vi "OuputMixer5782_1Ghz_interpolated_single_cycle.vi"(6 "Standard interp":bool=TRUE, 7 "reset":bool, 8 "input valid":bool=TRUE, 9 "Sine in":fxp<+/-,16,0>[](array[numeric])=[0.0, 0.0, 0.0, 0.0], 10 "Cosine in":fxp<+/-,16,0>[](array[numeric])=[0.0, 0.0, 0.0, 0.0], 11 "Data":fxp<+/-,16,14>[](array[numeric])=[0.0, 0.0]) -> (3 "test":i16[](array[numeric]))   [LabVIEW 2018]
doc: "Outputs input from channel 0 as I*cos(t)-Q*sin(t) on analog output 0"
uses:
  <vilib>/rvi/eio/common/nirviEmuTemplateMethod_errors.vi
  <vilib>/eio/EIONode/EIONode.xnode
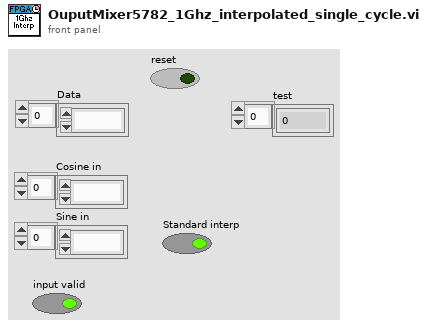
[diagram p1: front panel]
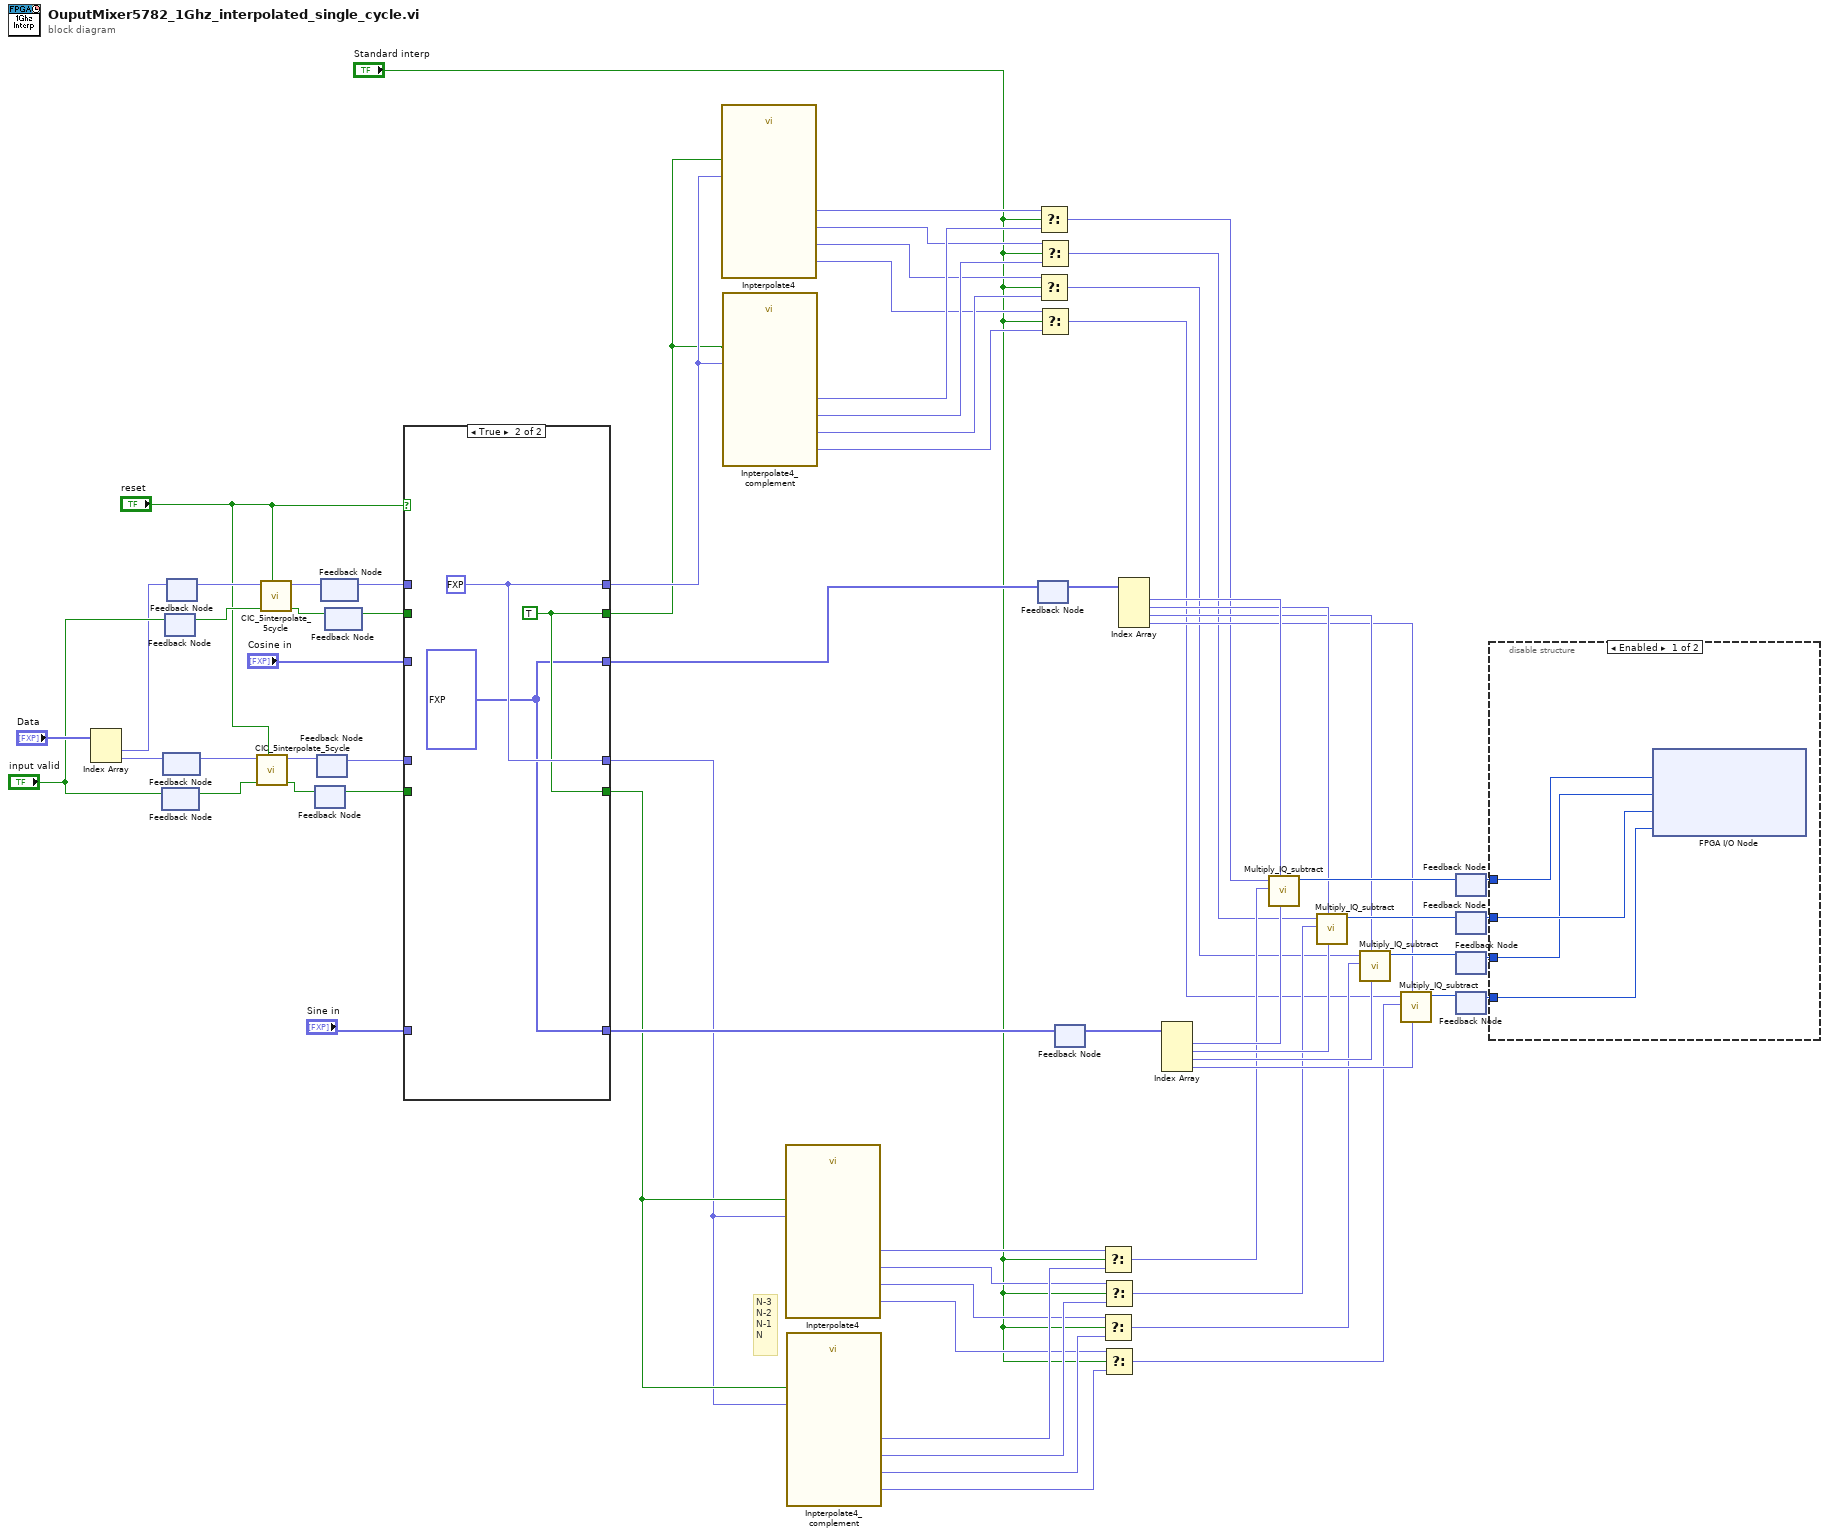
[diagram p0: block diagram]
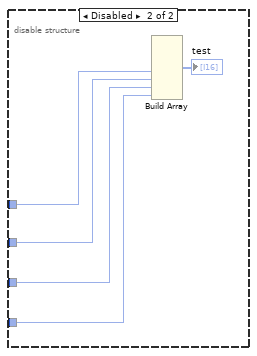
[diagram p3: hidden frame]
diagram:
  # "N-3\nN-2\nN-1\nN"
  n1 = Index Array(array="Data") -> (element #1=w46:fxp<+/-,16,14>, element #2=w47:fxp<+/-,16,14>)  [unwired: 2 in]
  n2 = feedback #1() -> (w54:bool)  [unwired: 1 in]
  n3 = feedback-in #1("input valid") -> ()
  n4 = feedback #2() -> (w56:fxp<+/-,16,14>)  [unwired: 1 in]
  n5 = feedback-in #2(w47) -> ()
  n6 = feedback #3() -> (w55:bool)  [unwired: 1 in]
  n7 = feedback-in #3("input valid") -> ()
  n8 = feedback #4() -> (w57:fxp<+/-,16,14>)  [unwired: 1 in]
  n9 = feedback-in #4(w46) -> ()
  n10 = call "CIC_5interpolate_5cycle.vi"("reset"="reset", "valid in"=w54, "Data in"=w56) -> ("valid out"=w48:bool, "Data out"=w53:fxp<+/-,16,14>)  [unwired: 7 in]
  n11 = call "CIC_5interpolate_5cycle.vi"("reset"="reset", "valid in"=w55, "Data in"=w57) -> ("valid out"=w49:bool, "Data out"=w52:fxp<+/-,16,14>)  [unwired: 7 in]
  n12 = feedback #5() -> (w35:bool)  [unwired: 1 in]
  n13 = feedback-in #5(w48) -> ()
  n14 = feedback #6() -> (w36:fxp<+/-,16,14>)  [unwired: 1 in]
  n15 = feedback-in #6(w53) -> ()
  n16 = feedback #7() -> (w32:fxp<+/-,16,14>)  [unwired: 1 in]
  n17 = feedback-in #7(w52) -> ()
  n18 = feedback #8() -> (w31:bool)  [unwired: 1 in]
  n19 = feedback-in #8(w49) -> ()
  n20 = case shown="True" "reset" {
    tunnel: [w71 w75] -> w66
    tunnel: w32 -> [w70 _]
    tunnel: "Cosine in" -> [w71 _]
    tunnel: w36 -> [w74 _]
    tunnel: [w74 w77] -> w28
    tunnel: w35 -> [w73 _]
    tunnel: [w73 w76] -> w29
    tunnel: "Sine in" -> [w72 _]
    tunnel: [w72 w75] -> w33
    tunnel: [w70 w77] -> w7
    tunnel: w31 -> [w69 _]
    tunnel: [w69 w76] -> w6
    frame False {
    }
    frame True {
      w75 = fxp<+/-,16,0>[] [0.0, 0.0, 0.0, 0.0] ("Cosine in")
      w76 = TRUE ("valid out")
      w77 = fxp<+/-,16,14> 0.0 ("Data out")
    }
  }
  n21 = call "Inpterpolate4.vi"("X"=w7, "input valid"=w6) -> ("X(t)"=w8:fxp<+/-,16,14>, "X(t -1)"=w9:fxp<+/-,16,14>, "X(t -2)"=w10:fxp<+/-,16,14>, "X(t -3)"=w11:fxp<+/-,16,14>)  [unwired: 9 in, 1 out]
  n22 = call "Inpterpolate4_complement.vi"("X"=w7, "input valid"=w6) -> ("X(t)"=w15:fxp<+/-,16,14>, "X(t -1)"=w13:fxp<+/-,16,14>, "X(t -2)"=w12:fxp<+/-,16,14>, "X(t -3)"=w14:fxp<+/-,16,14>)  [unwired: 9 in, 1 out]
  n23 = call "Inpterpolate4.vi"("X"=w28, "input valid"=w29) -> ("X(t)"=w16:fxp<+/-,16,14>, "X(t -1)"=w17:fxp<+/-,16,14>, "X(t -2)"=w18:fxp<+/-,16,14>, "X(t -3)"=w19:fxp<+/-,16,14>)  [unwired: 9 in, 1 out]
  n24 = call "Inpterpolate4_complement.vi"("X"=w28, "input valid"=w29) -> ("X(t)"=w27:fxp<+/-,16,14>, "X(t -1)"=w23:fxp<+/-,16,14>, "X(t -2)"=w22:fxp<+/-,16,14>, "X(t -3)"=w24:fxp<+/-,16,14>)  [unwired: 9 in, 1 out]
  n25 = feedback #9() -> (w67:fxp<+/-,16,0>[])  [unwired: 1 in]
  n26 = feedback-in #9(w66) -> ()
  n27 = Select(t=w11, s="Standard interp", f=w14) -> (s? t:f=w5:fxp<+/-,16,14>)
  n28 = Select(t=w9, s="Standard interp", f=w13) -> (s? t:f=w3:fxp<+/-,16,14>)
  n29 = Select(t=w10, s="Standard interp", f=w12) -> (s? t:f=w4:fxp<+/-,16,14>)
  n30 = Select(t=w8, s="Standard interp", f=w15) -> (s? t:f=w2:fxp<+/-,16,14>)
  n31 = feedback #10() -> (w68:fxp<+/-,16,0>[])  [unwired: 1 in]
  n32 = feedback-in #10(w33) -> ()
  n33 = Select(t=w19, s="Standard interp", f=w24) -> (s? t:f=w20:fxp<+/-,16,14>)
  n34 = Select(t=w17, s="Standard interp", f=w23) -> (s? t:f=w25:fxp<+/-,16,14>)
  n35 = Select(t=w18, s="Standard interp", f=w22) -> (s? t:f=w21:fxp<+/-,16,14>)
  n36 = Select(t=w16, s="Standard interp", f=w27) -> (s? t:f=w26:fxp<+/-,16,14>)
  n37 = Index Array(array=w67) -> (element #1=w45:fxp<+/-,16,0>, element #2=w40:fxp<+/-,16,0>, element #3=w39:fxp<+/-,16,0>, element #4=w38:fxp<+/-,16,0>)  [unwired: 4 in]
  n38 = Index Array(array=w68) -> (element #1=w44:fxp<+/-,16,0>, element #2=w43:fxp<+/-,16,0>, element #3=w42:fxp<+/-,16,0>, element #4=w41:fxp<+/-,16,0>)  [unwired: 4 in]
  n39 = call "Multiply_IQ_subtract.vi"("Sin"=w44, "Cos"=w45, "Q"=w20, "I"=w5) -> ("Z"=w65:i16)  [unwired: 6 in, 1 out]
  n40 = call "Multiply_IQ_subtract.vi"("Sin"=w43, "Cos"=w40, "Q"=w21, "I"=w4) -> ("Z"=w64:i16)  [unwired: 6 in, 1 out]
  n41 = call "Multiply_IQ_subtract.vi"("Sin"=w42, "Cos"=w39, "Q"=w25, "I"=w3) -> ("Z"=w63:i16)  [unwired: 6 in, 1 out]
  n42 = call "Multiply_IQ_subtract.vi"("Sin"=w41, "Cos"=w38, "Q"=w26, "I"=w2) -> ("Z"=w62:i16)  [unwired: 6 in, 1 out]
  n43 = feedback #11() -> (w61:i16)  [unwired: 1 in]
  n44 = feedback-in #11(w65) -> ()
  n45 = feedback #12() -> (w60:i16)  [unwired: 1 in]
  n46 = feedback-in #12(w64) -> ()
  n47 = feedback #13() -> (w59:i16)  [unwired: 1 in]
  n48 = feedback-in #13(w63) -> ()
  n49 = feedback #14() -> (w58:i16)  [unwired: 1 in]
  n50 = feedback-in #14(w62) -> ()
  n51 = disable-structure shown="Enabled" {
    disable-tunnel: w61 -> [w81 w86]
    disable-tunnel: w60 -> [w80 w85]
    disable-tunnel: w59 -> [w79 w84]
    disable-tunnel: w58 -> [w78 w83]
    frame Enabled {
      n52 = xnode "FPGA I/O Node"("IO Module\\AO 0 N-1"=w81, "IO Module\\AO 0 N"=w79, "IO Module\\AO 1 N-1"=w80, "IO Module\\AO 1 N"=w78) -> ()  [unwired: 4 in, 4 out]
    }
    frame Disabled {
      n53 = Build Array(w86, w85, w84, w83) -> (→"test":i16[], w90:i16, w89:i16, w88:i16, w87:i16)
    }
  }
